vi "LandmarkNavigator.vi"(7 "Score cutoff":dbl, 8 "error in":errorcluster, 9 "Color Components":T2={"Hue"={110.0, 142.0}, "Sat"={138.0, 255.0}, "Val"={139.0, 198.0}} {"Val" scale=0.0..255.0; "Sat" scale=0.0..255.0; "Hue" scale=0.0..255.0 scale format="%#_3g"}, 10 "Color System":u16(ring)=2 items=["RGB", "HSL", "HSV", "HSI"], 11 "Image":T1) -> (0 "error out":errorcluster, 3 "Image out":T1)   [LabVIEW 2013]
doc: "Determines if the goal is hot or not and returns an enum to indicate this. Also returns the calculated distance to the goal."
uses:
  <vilib>/vision/Image Controls.llb/IMAQ Image.ctl
  Example_Code/2014 Target Detection/TargetType.ctl
panel:
  in  "Camera Type":enum16{"206", "1011", "1013"}(ring)=enum."1013"
  in  "Area Size Limit %":dbl=0.06 format="%#_13g"
  out "Mask":T1(plugin-control)
  out "Image":T1(plugin-control)
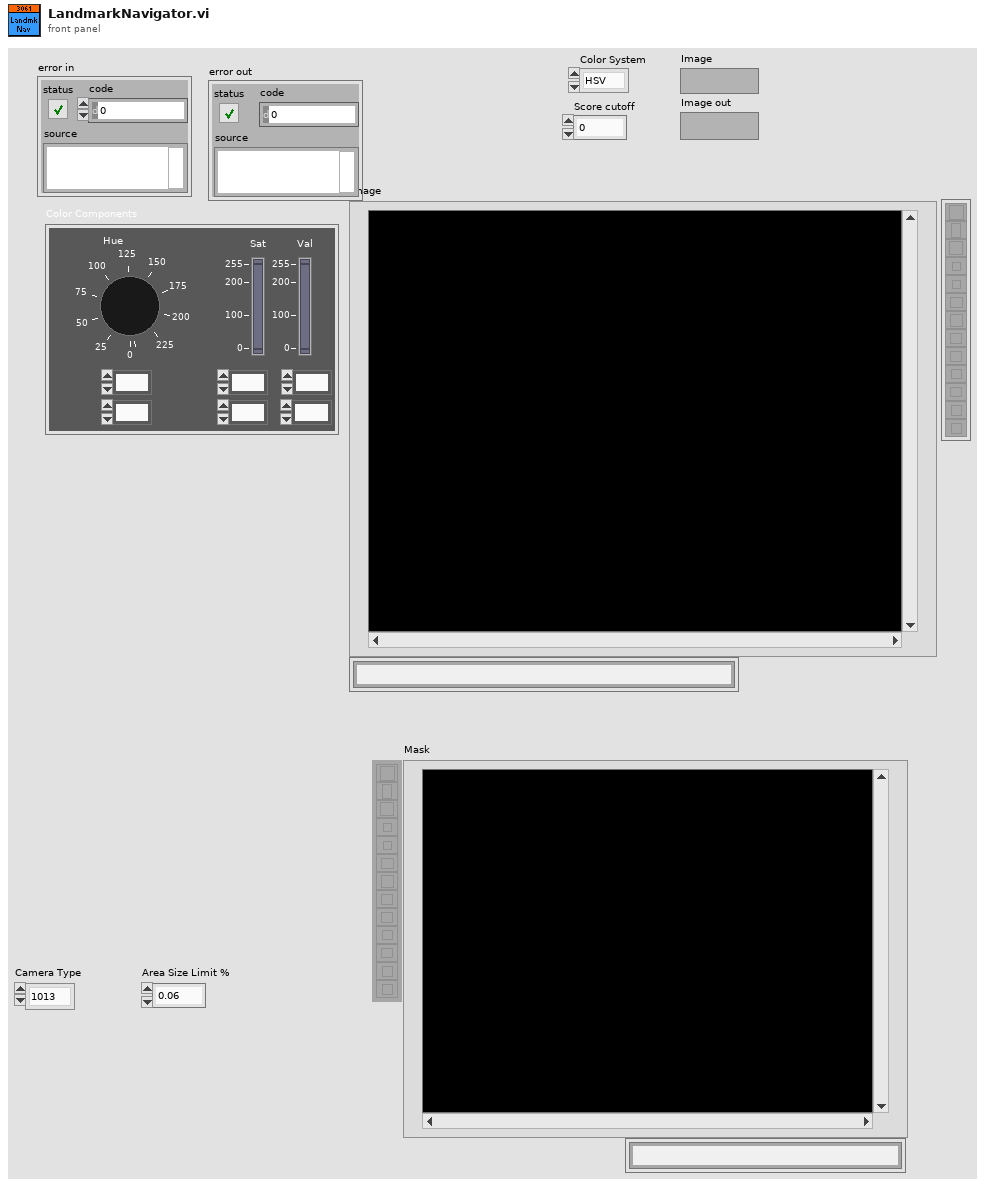
[diagram p1: front panel]
types:
  T1 = typedef "IMAQ Image.ctl" = refnum<image>
  T2 = cluster{"Hue":cluster{dbl, dbl}, "Sat":cluster{dbl, dbl}, "Val":cluster{dbl, dbl}}
  T3 = typedef "TargetType.ctl" = enum16{"Not Hot", "Hot"}
  T4 = cluster{"Distance (ft)":dbl, "Target Center (-1 to 1)":cluster{"X":dbl, "Y":dbl}, bool, "State":T3, "Target Center (Angles)":cluster{dbl, dbl}, "Center Displacement (ft)":dbl}
  T5 = cluster{"Horizontal":bool, "Aspect Score":dbl, "Rect Score":dbl, cluster{"Left":dbl, "Top":dbl, "Right":dbl, "Bottom":dbl}, "Equiv H":dbl, "Equiv V":dbl}[]
  T6 = cluster{"Scores":cluster{"Total":dbl, "Left":dbl, "Right":dbl, "Ratio":dbl, "Vertical":dbl, "index":i32, "State":T3}, "Verticals":cluster{"Horizontal?":bool, "Aspect Score":dbl, "Rect Score":dbl, cluster{"Left":dbl, "Top":dbl, "Right":dbl, "Bottom":dbl}, "Equiv H":dbl, "Equiv V":dbl}, "Horizontals":cluster{"Horizontal?":bool, "Aspect Score":dbl, "Rect Score":dbl, cluster{"Left":dbl, "Top":dbl, "Right":dbl, "Bottom":dbl}, "Equiv H":dbl, "Equiv V":dbl}, "Validated":bool}[]
  T7 = cluster{"Distance (ft)":dbl, "Target Center (-1 to 1)":cluster{"X":dbl, "Y":dbl}, bool, "State":T3, "Target Center (Angles)":cluster{dbl, dbl}, "Center Displacement (ft)":dbl}[]
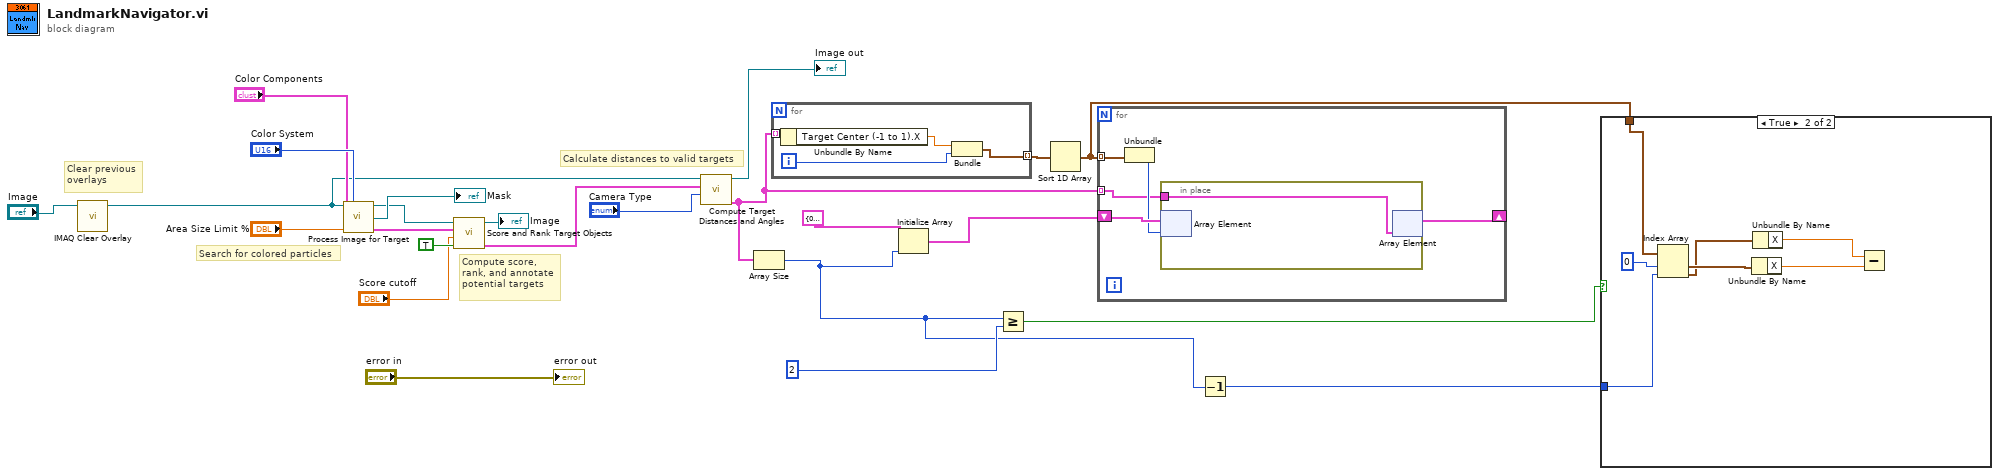
[diagram p0: block diagram]
diagram:
  # "Calculate distances to valid targets"
  # "Clear previous\noverlays"
  # "Search for colored particles"
  # "Compute score,\nrank, and annotate\npotential targets"
  n1 = call "IMAQ Clear Overlay"("Image"="Image") -> ("Image Out"=w12:T1)  [unwired: 9 in, 1 out]
  n2 = call "Process Image for Target.vi"("Src Image"=w12, "Color Mode"="Color System", "Color Components"="Color Components", "Area Cutoff %"="Area Size Limit %") -> ("Src Image Out"=w22:T1, "Threshold"=→"Mask":T1, "Particles"=w20:T5)  [unwired: 9 in]
  n3 = call "Score and Rank Target Objects.vi"("Annotate"=TRUE, "Score Limit"="Score cutoff", "Particles"=w20, "Image in"=w22) -> ("Target Info"=w13:T6, "Annotated Image"=→"Image":T1)  [unwired: 6 in]
  n4 = call "Compute Target Distances and Angles.vi"("Camera Type"="Camera Type", "Target Info"=w13, "Image in"=w12) -> ("Distances"=w4:T7, "Image out"=→"Image out":T1)  [unwired: 6 in, 1 out]
  n5 = Array Size(array=w4) -> (size(s)=w2:i32)
  n6 = for {
    tunnel: w4 -> [w28] mode=indexing
    tunnel: [w25] -> w5 mode=indexing
    i -> [w26]
    n7 = Unbundle By Name(w28) -> ("Target Center (-1 to 1).X"=w27:dbl)
    n8 = Bundle("X"=w27, w26) -> (w25:cluster{"X":dbl, i32})  [unwired: 1 in]
  }
  n9 = Initialize Array(T4 {"Distance (ft)"=0.0, "Target Center (-1 to 1)"={"X"=0.0, "Y"=0.0}, FALSE, "State"=enum."Not Hot", "Target Center (Angles)"={0.0, 0.0}, "Center Displacement (ft)"=0.0}, w2) -> (w6:T7)
  n10 = Greater Or Equal?(x=w2, y=2) -> (x >= y?=w9:bool)
  n11 = Sort 1D Array(array=w5) -> (sorted array=w3:cluster{"X":dbl, i32}[])
  n12 = for {
    shift-right: [w32] -> _
    shift-left: w6 -> [w33]
    tunnel: w3 -> [w31] mode=indexing
    tunnel: w4 -> [w29] mode=indexing
    n13 = Unbundle(w31) -> (w30:i32)  [unwired: 1 out]
    n14 = in-place {
      in-place-border: w29 -> [w34]
      n15 = in-place-array #1(w33, w30) -> ()  [unwired: 1 out]
      n16 = in-place-array #1(w34) -> (w32:T7)  [unwired: 1 out]
    }
  }
  n17 = Decrement(x=w2) -> (x-1=w1:i32)
  n18 = case shown="True" w9 {
    tunnel: w3 -> [_ w39]
    tunnel: w1 -> [_ w38]
    frame False {
    }
    frame True {
      n19 = Index Array(array=w39, index #1=0 ("index"), index #2=w38) -> (element #1=w40:cluster{"X":dbl, i32}, element #2=w37:cluster{"X":dbl, i32})
      n20 = Unbundle By Name(w40) -> ("X"=w36:dbl)
      n21 = Unbundle By Name(w37) -> ("X"=w35:dbl)
      n22 = Subtract(x=w35, y=w36) -> ()  [unwired: 1 out]
    }
  }
  "error out" <- "error in"
